vi "4. Main.vi"() -> ()   [LabVIEW 2014, in "Hello World - Introduction to Widgets.lvlib"]
doc: "Copyright (c) 2016 Sze Howe Koh\nThis code is licensed under the MIT license"
uses:
  Hello World - Introduction to Widgets.lvlib
  src/LabVIEW/LQ Core/QSize.ctl
  src/LabVIEW/Qt Widgets/QWidget/resize.vi
  src/LabVIEW/Qt Widgets/QWidget/setVisible.vi
  src/LabVIEW/LQ Core/LQCoreEngine/LQCoreEngine.lvclass
  Number Widget/4. Number Widget.lvclass
panel:
  in  "Stop Button":bool
  # "Prerequisite knowledge/experience\n- Examples 1-3 in this series\n- LabVIEW object-oriented programming (http://www.ni.com/white-paper/3573/en/)\n\n\nDescription\nThis example takes the widget code from 3a. Connecting a Signal to a Qt Slot and encapsulates it in a\ndedicated LVClass called Number Widget.\n\nThere are a few reasons to do this:\n- To keep code organized. Notice that the block diagram for 4. Main.vi is simpler than 3a. Main.vi.\n- To inherit the features of existing widgets, without having to rewriting it from scratch.\n- To make it easy to re-use your custom widget code. See tutorial 6. Reusing Components Dynamically.\n\n(Note: Because tutorials 4 - 6 each have their own copy of Number Widget, they are prefixed with their\ntutorial numbers to avoid a naming conflict. This is generally not required, however.)\n\n\nShowcase\n- Inheritable GUI components"
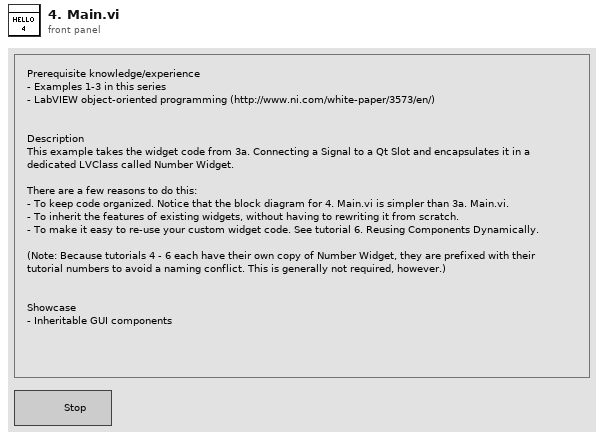
[diagram p1: front panel]
types:
  T1 = typedef "QSize.ctl" = cluster{"width":i32, "height":i32}
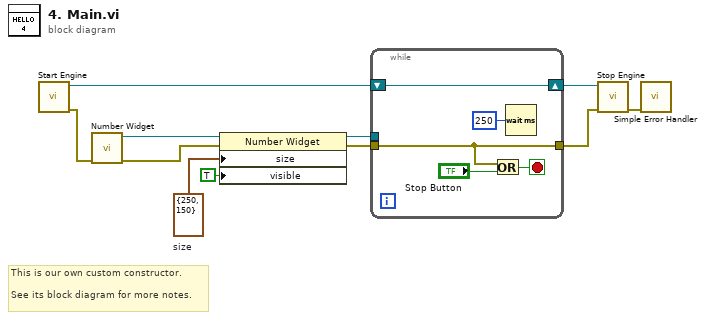
[diagram p0: block diagram]
diagram:
  w7 = T1 {"width"=250, "height"=150}  # size
  # "This is our own custom constructor.\n\nSee its block diagram for more notes."
  n1 = call "Start Engine.vi"() -> ("Error Out"=w2:errorcluster, "New Engine"=w11:refnum<class "LQCoreEngine.lvclass">)  [unwired: 10 in]
  n2 = call "Number Widget.vi"("Error In"=w2) -> ("Error Out"=w1:errorcluster, "New Number Widget"=w3:refnum<class "4. Number Widget.lvclass">)  [unwired: 9 in]
  n3 = property class="Number Widget"(reference=w3, error in=w1, "size"=w7, "visible"=TRUE) -> (reference out=w4:refnum<class "4. Number Widget.lvclass">, error out=w9:errorcluster)
  n4 = while {
    shift-right: [w16] -> w10
    shift-left: w11 -> [w16]
    tunnel: w9 -> [w12]
    tunnel: [w12] -> w5
    tunnel: w4 -> [_]
    stop <- w14 stop-if-true
    n5 = Or(x=w12, y="Stop Button") -> (x .or. y?=w14:bool)
    n6 = Wait (ms)(milliseconds to wait=u32 250) -> ()  [unwired: 1 out]
  }
  n7 = call "Stop Engine.vi"("Error In"=w5, "LQCoreEngine"=w10) -> ("Error Out"=w8:errorcluster)  [unwired: 9 in]
  n8 = call <vilib>:"Simple Error Handler.vi"("error in (no error)"=w8) -> ()  [unwired: 4 in, 5 out]
